vi "SDCP Receiver and Transmitter - Obtain data bytes.vi"(2 "error in (no error)":errorcluster, 3 "Table element in":T1={"Frame ID"=0, "Frame Name"="", "Data Bytes"=[], "Cycle time (ms)"=0, "Counter"=0, "Trigger mode"=enum."Cyclic", "Trigger state"=enum."Start cyclic trigger", "Parameter names"=[], "Parameter values"=[]}) -> (0 "error out":errorcluster, 1 "Table element out":T1={"Frame ID"=0, "Frame Name"="", "Data Bytes"=[], "Cycle time (ms)"=0, "Counter"=0, "Trigger mode"=enum."Cyclic", "Trigger state"=enum."Start cyclic trigger", "Parameter names"=[], "Parameter values"=[]})   [LabVIEW 2020]
uses:
  Typedefs/SDCP SMF Receiver and Transmitter - Transmit Table Element.ctl
  Typedefs/SDCP - Standard Message Frame Parameters - FGV - commands.ctl
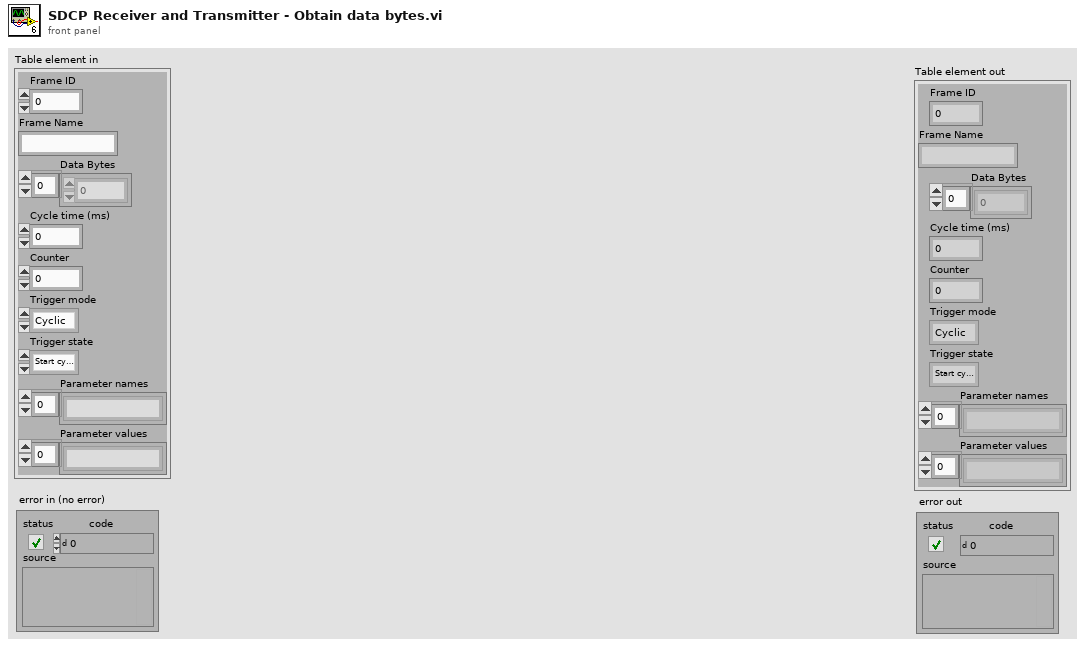
[diagram p1: front panel]
types:
  T1 = typedef "SDCP SMF Receiver and Transmitter - Transmit Table Element.ctl" = cluster{"Frame ID":i32, "Frame Name":string, "Data Bytes":u8[], "Cycle time (ms)":i32, "Counter":i32, "Trigger mode":enum16{"Triggered", "Cyclic"}, "Trigger state":enum16{"Stop cyclic trigger", "Start cyclic trigger", "Stop single trigger", "Start single trigger"}, "Parameter names":string[], "Parameter values":string[]}
  T2 = typedef "SDCP - Standard Message Frame Parameters - FGV - commands.ctl" = enum16{"Write descriptors", "Read descriptors", "Read values", "Load parameters from file", "Write values", "Read all descriptors"}
  T3 = typedef "SDCP - SMF parameter descriptors.ctl" = cluster{"Frame name":string, "Frame ID":i32, "Data type":string, "Start Position":i32, "Length":i32, "Factor":dbl, "Offset":dbl, "Parameter name":string, "Value":string}
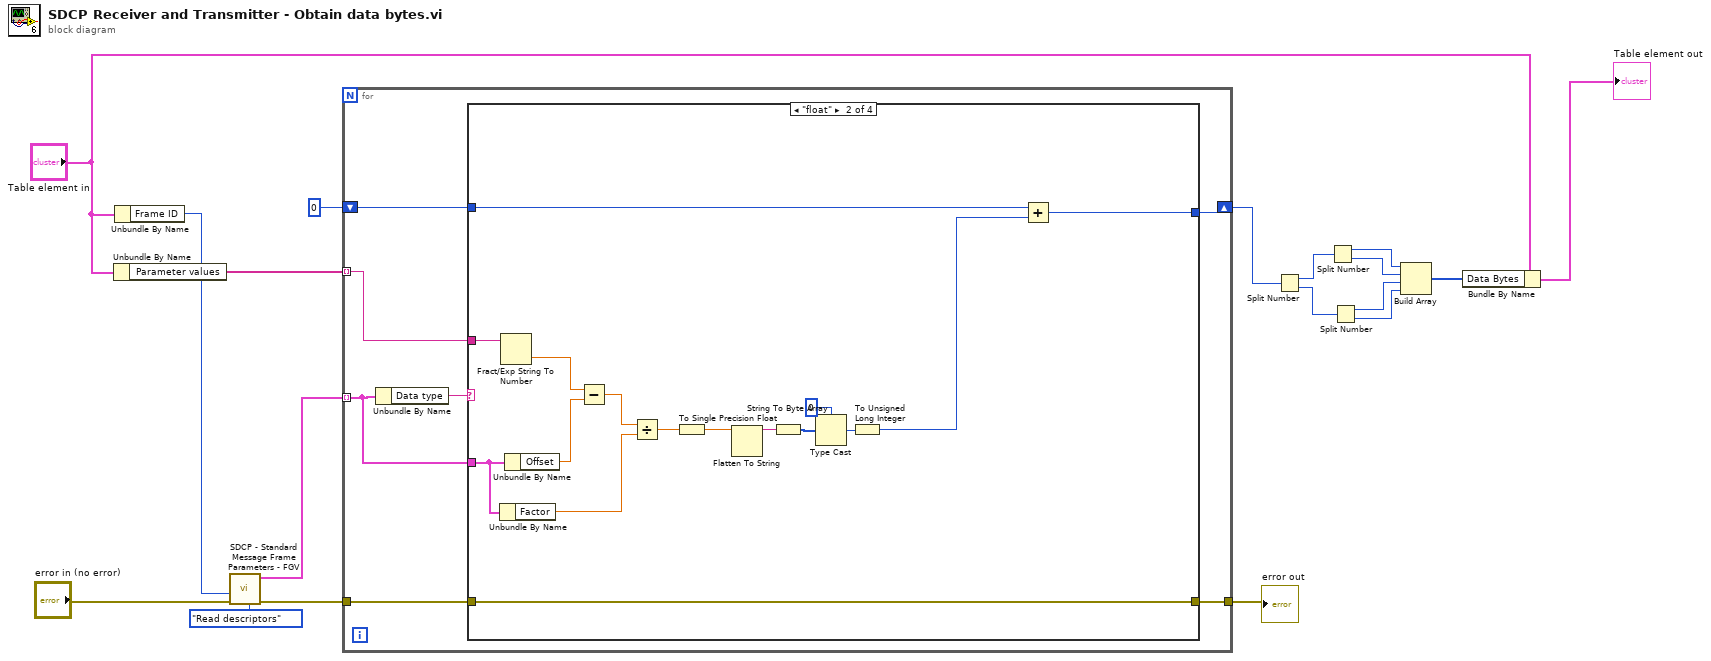
[diagram p0: block diagram]
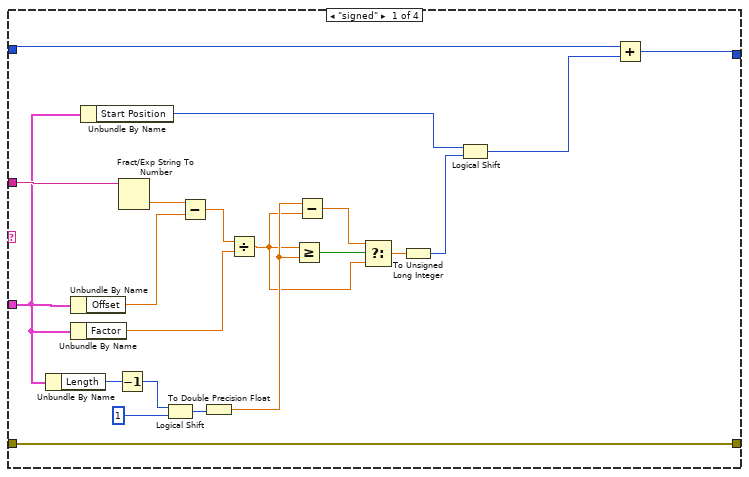
[diagram p2: hidden frame]
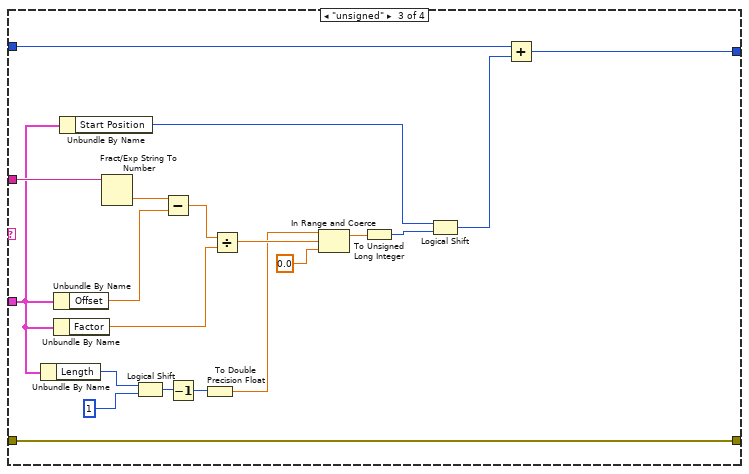
[diagram p3: hidden frame]
diagram:
  n1 = Unbundle By Name("Table element in") -> ("Parameter values"=w13:string[])
  n2 = Unbundle By Name("Table element in") -> ("Frame ID"=w16:i32)
  n3 = call "SDCP - Standard Message Frame Parameters - FGV.vi"("FID"=w16, "error in (no error)"="error in (no error)", "Command"=SDCP_-_Standard_Message_Frame_Parameters_-_FGV_-_commands."Read descriptors") -> ("SMF Parameters descriptors out"=w14:T3[], "error out"=w15:errorcluster)  [unwired: 4 in]
  n4 = for {
    tunnel: w15 -> [w20]
    tunnel: w14 -> [w23] mode=indexing
    tunnel: w13 -> [w24] mode=indexing
    shift-right: [w21] -> w10
    shift-left: u32 0 -> [w22]
    tunnel: [w19] -> w11
    n5 = Unbundle By Name(w23) -> ("Data type"=w25:string)
    n6 = case shown="\"float\"" w25 {
      tunnel: w24 -> [w42 w62 w82 _]
      tunnel: w23 -> [w32 w58 w70 _]
      tunnel: w22 -> [w28 w50 w68 w84]
      tunnel: [w27 w48 w64 w84] -> w21
      tunnel: w20 -> [w26 w47 w63 w83]
      tunnel: [w26 w47 w63 w83] -> w19
      frame "signed" {
        n7 = Unbundle By Name(w32) -> ("Length"=w41:i32)
        n8 = Unbundle By Name(w32) -> ("Offset"=w45:dbl)
        n9 = Unbundle By Name(w32) -> ("Factor"=w43:dbl)
        n10 = Unbundle By Name(w32) -> ("Start Position"=w31:i32)
        n11 = Decrement(x=w41) -> (x-1=w40:i32)
        n12 = Fract/Exp String To Number(string=w42) -> (number=w46:dbl)  [unwired: 3 in, 1 out]
        n13 = Logical Shift(y=w40, x=u32 1) -> (x << y=w38:u32)
        n14 = Subtract(x=w46, y=w45) -> (x-y=w44:dbl)
        n15 = To Double Precision Float(number=w38) -> (double precision float=w35:dbl)
        n16 = Divide(x=w44, y=w43) -> (x/y=w34:dbl)
        n17 = Greater Or Equal?(x=w34, y=w35) -> (x >= y?=w37:bool)
        n18 = Subtract(x=w35, y=w34) -> (x-y=w36:dbl)
        n19 = Select(t=w36, s=w37, f=w34) -> (s? t:f=w33:dbl)
        n20 = To Unsigned Long Integer(number=w33) -> (unsigned 32bit integer=w30:u32)
        n21 = Logical Shift(y=w31, x=w30) -> (x << y=w29:u32)
        n22 = Add(x=w28, y=w29) -> (x+y=w27:u32)
      }
      frame "float" {
        n23 = Unbundle By Name(w58) -> ("Factor"=w57:dbl)
        n24 = Fract/Exp String To Number(string=w62) -> (number=w61:dbl)  [unwired: 3 in, 1 out]
        n25 = Unbundle By Name(w58) -> ("Offset"=w60:dbl)
        n26 = Subtract(x=w61, y=w60) -> (x-y=w59:dbl)
        n27 = Divide(x=w59, y=w57) -> (x/y=w56:dbl)
        n28 = To Single Precision Float(number=w56) -> (single precision float=w51:sgl)
        n29 = Flatten To String(anything=w51) -> (data string=w55:string)  [unwired: 3 in, 2 out]
        n30 = String To Byte Array(string=w55) -> (unsigned byte array=w54:u8[])
        n31 = Type Cast(type=u32 0, x=w54) -> (*(type *) &x=w52:u32)
        n32 = To Unsigned Long Integer(number=w52) -> (unsigned 32bit integer=w49:u32)
        n33 = Add(x=w50, y=w49) -> (x+y=w48:u32)
      }
      frame "unsigned" {
        n34 = Unbundle By Name(w70) -> ("Length"=w77:i32)
        n35 = Unbundle By Name(w70) -> ("Offset"=w80:dbl)
        n36 = Unbundle By Name(w70) -> ("Factor"=w78:dbl)
        n37 = Unbundle By Name(w70) -> ("Start Position"=w69:i32)
        n38 = Fract/Exp String To Number(string=w82) -> (number=w81:dbl)  [unwired: 3 in, 1 out]
        n39 = Logical Shift(y=w77, x=u64 1) -> (x << y=w75:u64)
        n40 = Subtract(x=w81, y=w80) -> (x-y=w79:dbl)
        n41 = Decrement(x=w75) -> (x-1=w74:u64)
        n42 = To Double Precision Float(number=w74) -> (double precision float=w72:dbl)
        n43 = Divide(x=w79, y=w78) -> (x/y=w73:dbl)
        n44 = In Range and Coerce(upper limit=w72, x=w73, lower limit=0.0) -> (coerced(x)=w66:dbl)  [unwired: 1 out]
        n45 = To Unsigned Long Integer(number=w66) -> (unsigned 32bit integer=w65:u32)
        n46 = Logical Shift(y=w69, x=w65) -> (x << y=w67:u32)
        n47 = Add(x=w68, y=w67) -> (x+y=w64:u32)
      }
      frame Default {
      }
    }
  }
  "error out" <- w11
  n48 = Split Number(x=w10) -> (hi(x)=w9:u16, lo(x)=w8:u16)
  n49 = Split Number(x=w9) -> (hi(x)=w7:u8, lo(x)=w6:u8)
  n50 = Split Number(x=w8) -> (hi(x)=w5:u8, lo(x)=w4:u8)
  n51 = Build Array(w7, w6, w5, w4) -> (w2:u8[])
  n52 = Bundle By Name(cluster="Table element in", "Data Bytes"=w2) -> (→"Table element out":T1)
